vi "subReadVersionFile.vi"() -> (0 "error out":errorcluster, 2 "Step Types Version":string, 3 "TestStand Versions":string)   [LabVIEW 2015, in "veristand-steps-build-tools.lvlib"]
uses:
  veristand-steps-build-tools.lvlib
  <vilib>/Utility/config.llb/Read Key (String).vi
  <vilib>/Utility/config.llb/NI_LVConfig.lvlib
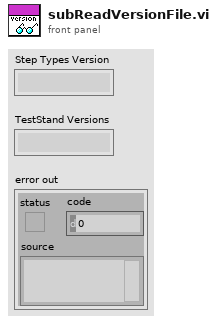
[diagram p1: front panel]
types:
  T1 = typedef "NI_LVConfig.lvlib/Config Data RefNum.ctl" = refnum<k1>
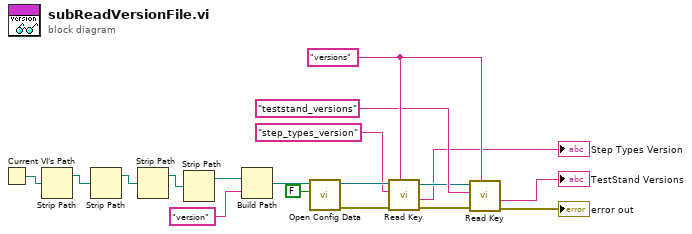
[diagram p0: block diagram]
diagram:
  w6 = "versions" ("section")
  n1 = Current VI's Path() -> (path=w18:path)
  n2 = Strip Path(path=w18) -> (stripped path=w17:path)  [unwired: 1 out]
  n3 = Strip Path(path=w17) -> (stripped path=w16:path)  [unwired: 1 out]
  n4 = Strip Path(path=w16) -> (stripped path=w14:path)  [unwired: 1 out]
  n5 = Strip Path(path=w14) -> (stripped path=w13:path)  [unwired: 1 out]
  n6 = Build Path(base path=w13, name or relative path="version") -> (appended path=w12:path)
  n7 = call <vilib>:"Open Config Data.vi"("create file if necessary (T)"=FALSE, "configuration file path"=w12) -> ("error out"=w9:errorcluster, "refnum"=w10:T1)  [unwired: 7 in, 1 out]
  n8 = call-poly <vilib>:"Read Key.vi"("section"=w6, "error in (no error)"=w9, "key"="step_types_version", "refnum"=w10) -> ("error out"=w7:errorcluster, "value"=→"Step Types Version":string, "refnum out"=w4:T1)  [unwired: 4 in, 1 out]
  n9 = call-poly <vilib>:"Read Key.vi"("section"=w6, "error in (no error)"=w7, "key"="teststand_versions", "refnum"=w4) -> ("error out"=→"error out":errorcluster, "value"=→"TestStand Versions":string)  [unwired: 4 in, 2 out]
